vi "Throw Error - Queue Already Exists.vi"(8 "Error In":errorcluster, 11 "Queue Name":string) -> (0 "Error Out":errorcluster)   [LabVIEW 2023, in "Anti-Spam Tester (AST).lvlib"]
doc: "Issues a command to the Process module by enqueuing into the Process module queue."
uses:
  Anti-Spam Tester (AST).lvlib
panel:
  # "Input\nInputs to the VI"
  # "Development\nControls or indicators that are useful for development or testing, but which are not outputs of the VI."
  # "Output\nOutputs of the VI"
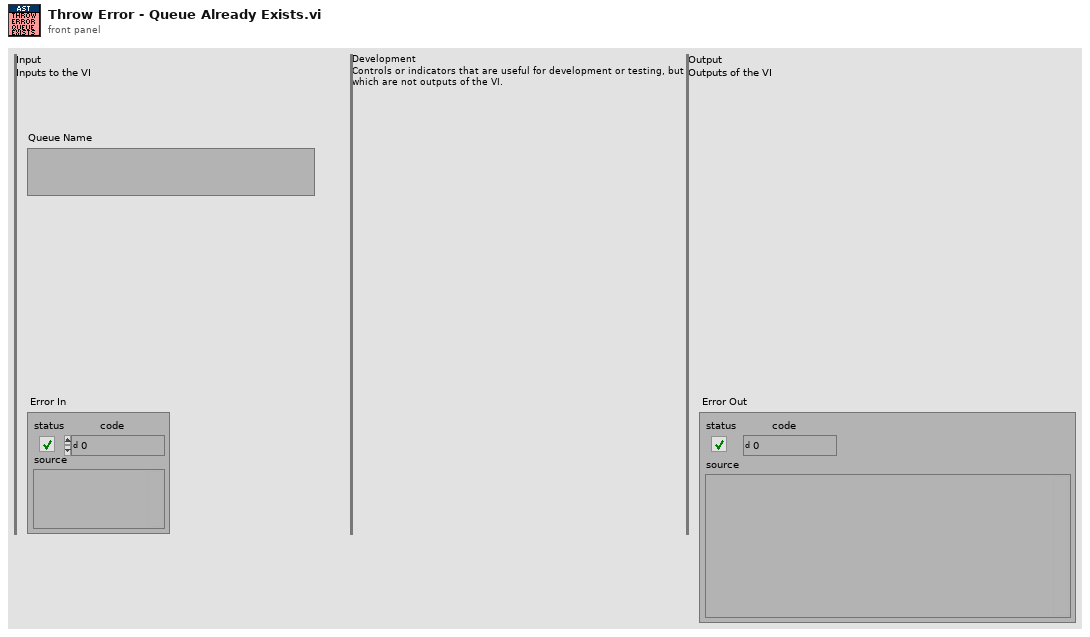
[diagram p1: front panel]
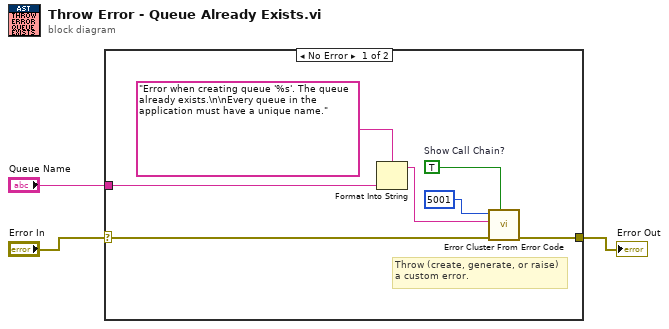
[diagram p0: block diagram]
diagram:
  n1 = case shown="No Error" "Error In" {
    selector: "Error In" -> [w7 w11]
    tunnel: [w6 w11] -> w2
    tunnel: "Queue Name" -> [w9 _]
    frame No Error {
      w4 = TRUE  # Show Call Chain?
      # "Throw (create, generate, or raise) a custom error."
      n2 = Format Into String(format string="Error when creating queue '%s'. The queue already exists.\n\nEvery queue in the application must have a unique name.", w9) -> (resulting string=w5:string)  [unwired: 2 in, 1 out]
      n3 = call <vilib>:"Error Cluster From Error Code.vi"(5:w4, 6:w7, 8:w5, 9:5001) -> (0:w6:errorcluster)  [unwired: 5 in]
    }
    frame Error {
      # "If error at input, do not overwrite."
    }
  }
  "Error Out" <- w2
